vi "Periodic Tasks.vi"(8 "error in":errorcluster) -> ()   [LabVIEW 2013]
doc: "This VI runs in parallel to other tasks. It can contain as many user-defined periodic loops as you need. These can carry out PID or other sorts of timed response."
uses:
  GroundPassWrapperStates.ctl
  RefnameEnum.ctl
  CollectorWrapAction.ctl
  DoubleSolenoidAction.ctl
  <vilib>/Rock Robotics/WPI/Compressor/WPI_CompressorGetSetRefNum.vi
  Robot Global Data.vi
  <vilib>/Rock Robotics/SystemInterfaces/Utilities/FPGA_UtilitiesLED Source.ctl
  <vilib>/Rock Robotics/SystemInterfaces/Utilities/FPGA_UtilitiesLED State.ctl
  SingleSolenoidAction.ctl
  TankDriveAction.ctl
  ShooterWrapperAction.ctl
  SonarAction.ctl
  AutoAlignMode.ctl
  CatchAction.ctl
panel:
  out "GroundWrapperIterations":i32=2743
  out "GroundPassWrapper":u32=50
  in  "CollectorMotorSpeed":dbl=1.0
  out "AutoDistanceWrapperIterations":i32=6512
  out "AutoDistanceWrapperTimer":u32=20
  in  "Slowdown":dbl=12.0 format="%#_13g"
  in  "Brake":dbl=6.0 format="%#_13g"
  in  "DesiredDistance":dbl=144.0 format="%#_13g"
  out "CatcherWrapperIterations":i32=2744
  out "CatcherWrapperTimer":u32=50
  out "CollectorWrapperTimer":u32=50
  out "CollectorWrapperIterations":i32=2743
  out "ShooterWrapperIterations":i32=2667
  out "ShooterWrapperTimer":u32=50
  out "CollectorIterations":i32=2737
  out "ClapperIterations":i32=2743
  out "RollerPneumaticIterations":i32=2743
  out "RollerMotorIterations":i32=2742
  out "FiringCylinderIterations":i32=2745
  out "KickerIterations":i32=2744
  out "SonicShifterIterations":i32=2744
  out "TankDriveIterations":i32=6485
  out "Collector Timer":u32=50
  out "Clapper Timer":u32=50
  out "Roller Pneumatic Timer":u32=50
  out "Firing Cylinder Timer":u32=50
  out "Sonic Shifter Timer":u32=50
  out "Kicker Timer":u32=50
  out "Roller Motor Timer":u32=51
  out "Tank Drive Timer":u32=21
  # "CATCH"
  # "SHOOTER WRAP"
  # "SONIC SHIFTER"
  # "TANK DRIVE"
  # "COLLECTOR WRAP"
  # "KICKER"
  # "ROLLER MOTOR"
  # "COLLECTOR ARM"
  # "FIRING CYLINDERS"
  # "AUTODISTANCE"
  # "ROLLER PNEUMATIC"
  # "CLAPPER"
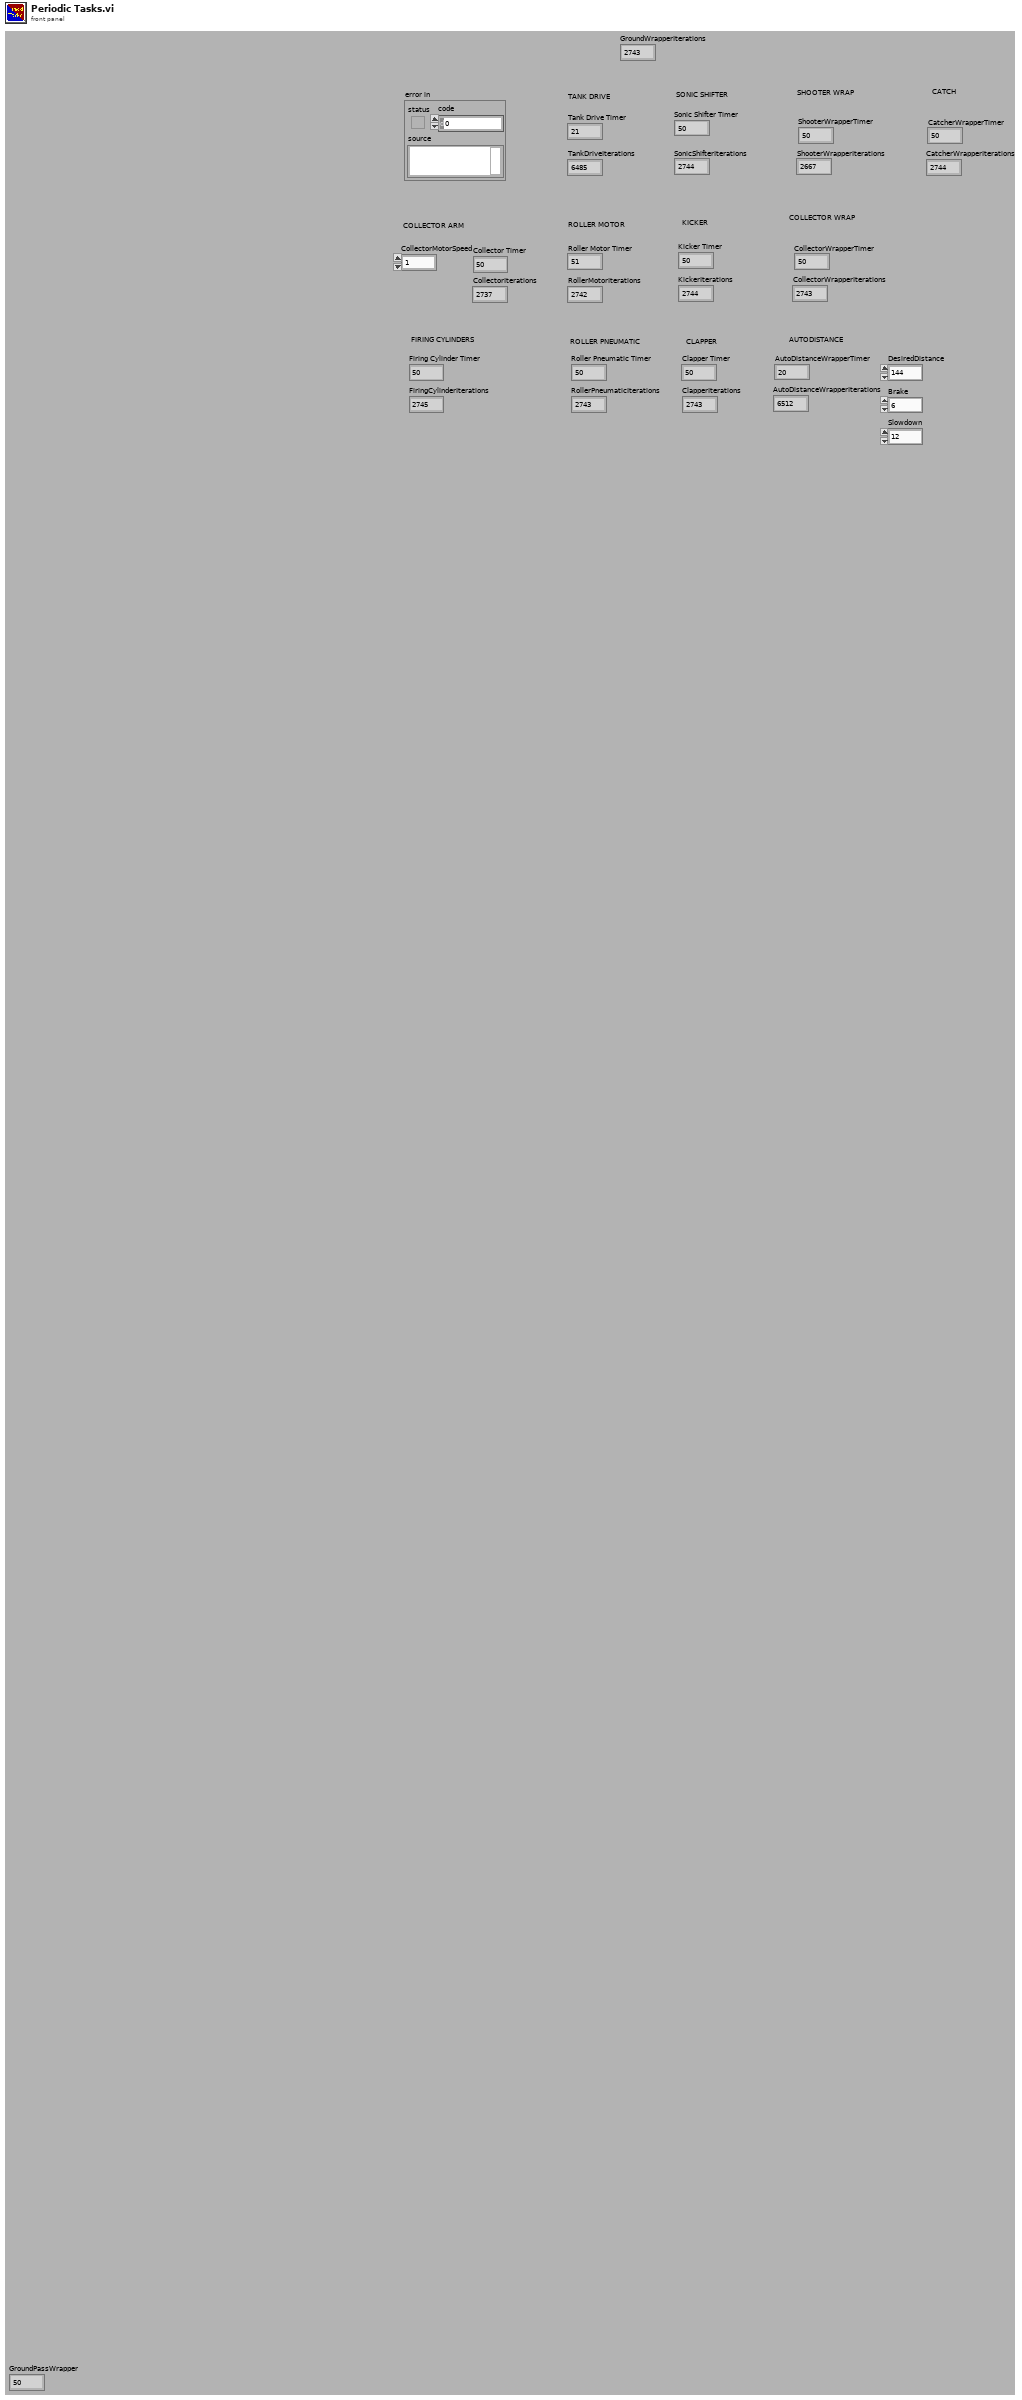
[diagram p1: front panel]
types:
  T1 = typedef "ShooterWrapperAction.ctl" = enum16{"Init", "CollectorDown", "CollectorUp"}
  T2 = typedef "CatchAction.ctl" = enum16{"PreCatch", "Catch", "Stop"}
  T3 = typedef "DoubleSolenoidAction.ctl" = enum16{"Init", "Middle", "In", "Out"}
  T4 = typedef "CollectorAction.ctl" = enum16{"Init", "Raise", "Lower", "Stop", "GetStatus"}
  T5 = typedef "CollectorWrapAction.ctl" = enum16{"PreCollect", "Collect", "Stop"}
  T6 = typedef "SingleSolenoidAction.ctl" = enum16{"Init", "SetState", "Disable"}
  T7 = typedef "TankDriveAction.ctl" = enum16{"Init", "LinearDrive", "SetValue", "Disable"}
  T8 = typedef "AutoAlignMode.ctl" = enum16{"Fullspeed", "Linear"}
  T9 = typedef "SonarAction.ctl" = enum16{"Init", "ReadValue", "Disable"}
  T10 = typedef "FPGA_UtilitiesLED State.ctl" = enum16{"Off", "On", "Toggle"}
  T11 = typedef "FPGA_UtilitiesLED Source.ctl" = enum16{"User LED", "FPGA LED"}
  T12 = typedef "RefnameEnum.ctl" = enum16{"TankDrive", "Controller1", "Controller2", "SonicShifter", "Compressor"}
  T13 = typedef "WPI_CompressorDevRef.ctl" = cluster{"DevStatus":errorcluster, "DigitalInputDevRef":T14, "RelayDevRef":T17}
  T14 = typedef "WPI_DigitalInputDevRef.ctl" = cluster{"DevStatus":errorcluster, "DIO Channel":T15, "Digital Module":T16}
  T15 = typedef "FPGA_DIOChannel.ctl" = enum8{"DIO 1", "DIO 2", "DIO 3", "DIO 4", "DIO 5", "DIO 6", "DIO 7", "DIO 8", "DIO 9", "DIO 10", "DIO 11", "DIO 12", "DIO 13", "DIO 14", "Invalid"}
  T16 = typedef "FPGA_TypedefDigitalModule.ctl" = enum16{"Digital Module 1", "Digital Module 2"}
  T17 = typedef "WPI_RelayDevRef.ctl" = cluster{"DevStatus":errorcluster, "Relay Channel":T18, "Digital Module":T16, "Relay Direction":T19}
  T18 = typedef "FPGA_DIORelayChannel.ctl" = enum8{"Relay 1", "Relay 2", "Relay 3", "Relay 4", "Relay 5", "Relay 6", "Relay 7", "Relay 8", "Invalid"}
  T19 = typedef "WPI_RelayDirection.ctl" = enum16{"Both directions", "Forward only", "Reverse only"}
  T20 = typedef "RollerAction.ctl" = enum16{"Init", "Off", "Forward", "Reverse"}
  T21 = typedef "GroundPassWrapperStates.ctl" = enum16{"Pass", "Stop"}
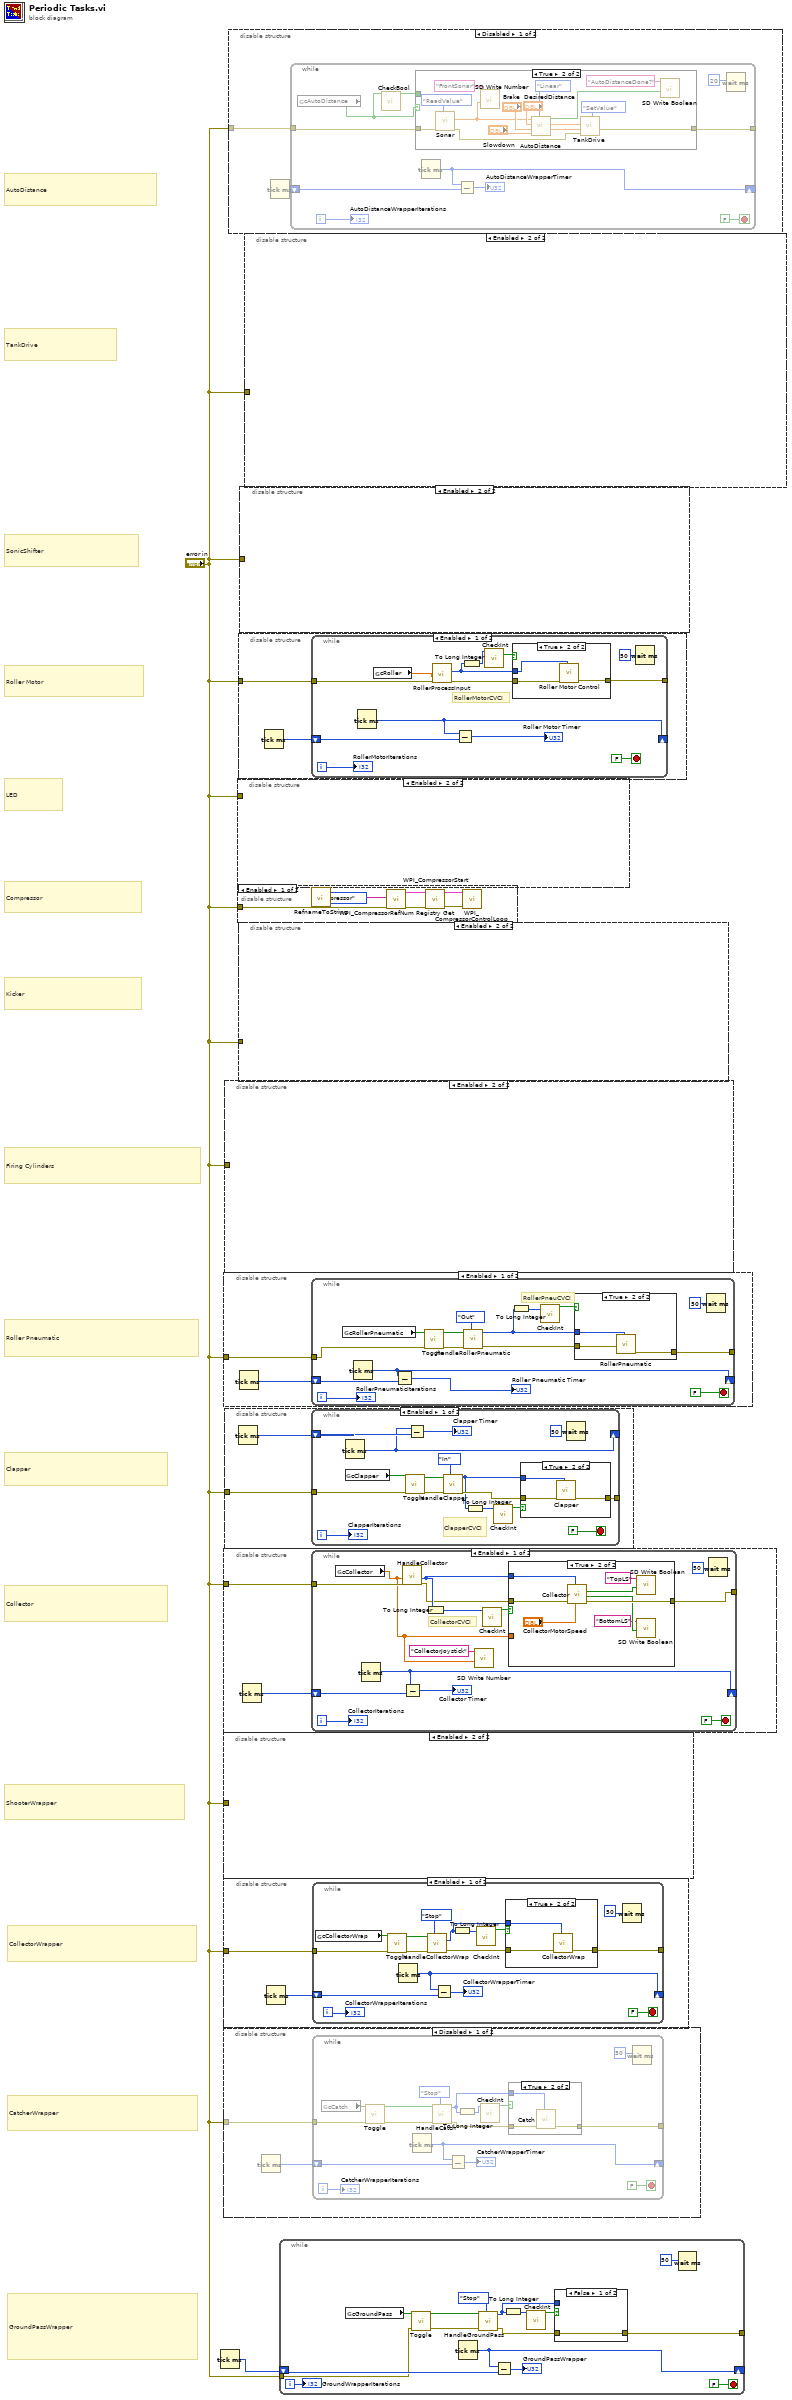
[diagram p0: block diagram]
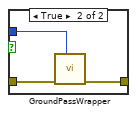
[diagram p2: hidden frame]
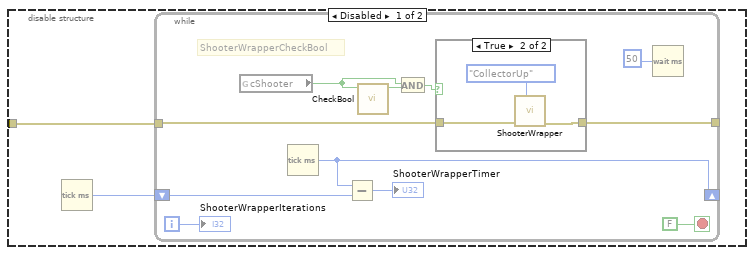
[diagram p7: hidden frame]
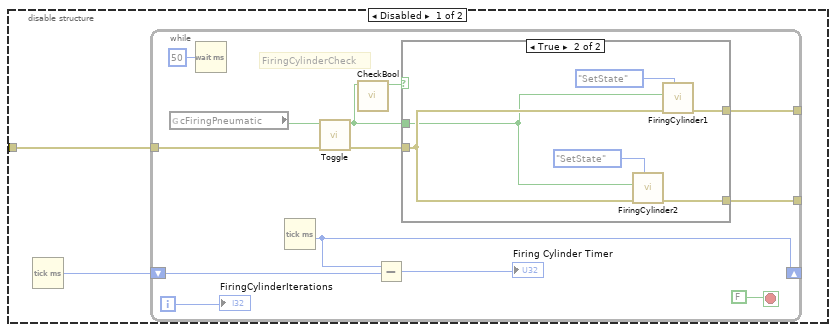
[diagram p15: hidden frame]
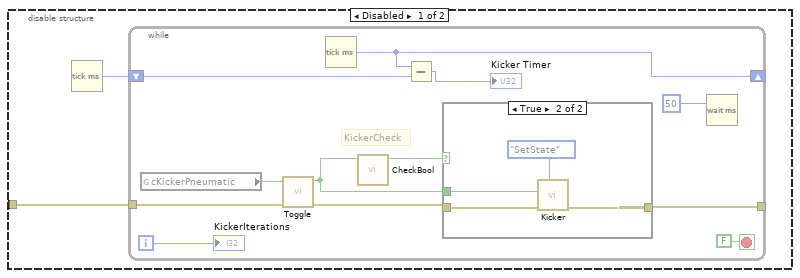
[diagram p17: hidden frame]
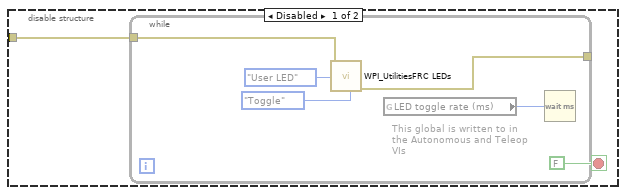
[diagram p20: hidden frame]
diagram:
  # "GroundPassWrapper"
  # "AutoDistance"
  # "CatcherWrapper"
  # "CollectorWrapper"
  # "ShooterWrapper"
  # "Collector"
  # "Clapper"
  # "Roller Pneumatic"
  # "Firing Cylinders"
  # "Kicker"
  # "Compressor"
  # "Roller Motor"
  # "SonicShifter"
  # "LED"
  # "TankDrive"
  n1 = Tick Count (ms)() -> (millisecond timer value=w1:u32)
  n2 = disable-structure shown="Enabled" {
    disable-tunnel: "error in" -> [w4 _]
    frame Disabled {
      n3 = Tick Count (ms)() -> (millisecond timer value=w3:u32)
      n4 = while {
        tunnel: w4 -> [w11]
        shift-right: [w12] -> _
        shift-left: w3 -> [w13]
        tunnel: [w10] -> _
        i -> [w8]
        stop <- FALSE stop-if-true
        # "ShooterWrapperCheckBool"
        n5 = global read "Robot Global Data.vi" "cShooter"() -> (w5:bool)
        n6 = Tick Count (ms)() -> (millisecond timer value=w12:u32)
        n7 = Subtract(x=w12, y=w13) -> (x-y=→"ShooterWrapperTimer":u32)
        n8 = call "CheckBool.vi"("Input Boolean"=w5) -> ("Boolean Changed?"=w7:bool)  [unwired: 10 in]
        n9 = And(x=w5, y=w7) -> (x .and. y?=w6:bool)
        n10 = case shown="True" w6 {
          tunnel: w11 -> [w16 w19]
          tunnel: [w16 w18] -> w10
          frame False {
          }
          frame True {
            n11 = call "ShooterWrapper.vi"("Action"=ShooterWrapperAction."CollectorUp", "error in"=w19) -> ("error out"=w18:errorcluster)  [unwired: 8 in]
          }
        }
        n12 = Wait (ms)(milliseconds to wait=u32 50) -> ()  [unwired: 1 out]
        "ShooterWrapperIterations" <- w8
      }
    }
    frame Enabled {
    }
  }
  n13 = disable-structure shown="Disabled" {
    disable-tunnel: "error in" -> [w21 _]
    frame Disabled {
      n14 = Tick Count (ms)() -> (millisecond timer value=w20:u32)
      n15 = while {
        tunnel: w21 -> [w37]
        tunnel: [w34] -> _
        shift-right: [w29] -> _
        shift-left: w20 -> [w30]
        i -> [w31]
        stop <- FALSE stop-if-true
        n16 = global read "Robot Global Data.vi" "cCatch"() -> (w36:bool)
        n17 = call "Toggle.vi"("error in"=w37, "RawInput"=w36) -> ("error out"=w27:errorcluster, "ToggleState"=w23:bool)  [unwired: 8 in]
        n18 = Tick Count (ms)() -> (millisecond timer value=w29:u32)
        n19 = call "HandleCatch.vi"("InitState"=CatchAction."Stop", "error in (no error)"=w27, "Toggle?"=w23) -> ("error out"=w26:errorcluster, "State"=w24:T2)  [unwired: 7 in]
        n20 = Subtract(x=w29, y=w30) -> (x-y=→"CatcherWrapperTimer":u32)
        n21 = To Long Integer(number=w24) -> (32bit integer=w25:i32)
        n22 = call "CheckInt.vi"("Integer"=w25) -> ("Changed?"=w35:bool)  [unwired: 10 in]
        n23 = case shown="True" w35 {
          tunnel: w26 -> [w38 w41]
          tunnel: [w38 w40] -> w34
          tunnel: w24 -> [_ w39]
          frame False {
          }
          frame True {
            n24 = call "Catch.vi"("Action"=w39, "error in (no error)"=w41) -> ("error out"=w40:errorcluster)  [unwired: 9 in]
          }
        }
        n25 = Wait (ms)(milliseconds to wait=u32 50) -> ()  [unwired: 1 out]
        "CatcherWrapperIterations" <- w31
      }
    }
    frame Enabled {
    }
  }
  n26 = disable-structure shown="Enabled" {
    disable-tunnel: "error in" -> [w43 _]
    frame Enabled {
      n27 = Tick Count (ms)() -> (millisecond timer value=w42:u32)
      n28 = while {
        tunnel: w43 -> [w47]
        shift-right: [w56] -> _
        shift-left: w42 -> [w55]
        tunnel: [w49] -> _
        i -> [w48]
        stop <- FALSE stop-if-true
        # "RollerPneuCVCI"
        n29 = global read "Robot Global Data.vi" "cRollerPneumatic"() -> (w45:bool)
        n30 = Tick Count (ms)() -> (millisecond timer value=w56:u32)
        n31 = Subtract(x=w56, y=w55) -> (x-y=→"Roller Pneumatic Timer":u32)
        n32 = call "Toggle.vi"("error in"=w47, "RawInput"=w45) -> ("error out"=w46:errorcluster, "ToggleState"=w44:bool)  [unwired: 8 in]
        n33 = call "HandleRollerPneumatic.vi"("InitState"=DoubleSolenoidAction."Out", "error in (no error)"=w46, "Toggle?"=w44) -> ("error out"=w50:errorcluster, "State"=w51:T3)  [unwired: 7 in]
        n34 = To Long Integer(number=w51) -> (32bit integer=w53:i32)
        n35 = call "CheckInt.vi"("Integer"=w53) -> ("Changed?"=w52:bool)  [unwired: 10 in]
        n36 = case shown="True" w52 {
          tunnel: w51 -> [_ w63]
          tunnel: w50 -> [w60 w62]
          tunnel: [w60 w61] -> w49
          frame False {
          }
          frame True {
            n37 = call "RollerPneumatic.vi"("State"=w63, "Error in"=w62) -> ("Error out"=w61:errorcluster)  [unwired: 9 in]
          }
        }
        n38 = Wait (ms)(milliseconds to wait=u32 50) -> ()  [unwired: 1 out]
        "RollerPneumaticIterations" <- w48
      }
    }
    frame Disabled {
    }
  }
  n39 = disable-structure shown="Enabled" {
    disable-tunnel: "error in" -> [w65 _]
    frame Enabled {
      n40 = Tick Count (ms)() -> (millisecond timer value=w64:u32)
      n41 = while {
        tunnel: w65 -> [w78]
        shift-right: [w75] -> _
        shift-left: w64 -> [w76]
        tunnel: [w69] -> _
        i -> [w68]
        stop <- FALSE stop-if-true
        # "CollectorCVCI"
        n42 = global read "Robot Global Data.vi" "cCollector"() -> (w66:dbl)
        n43 = Tick Count (ms)() -> (millisecond timer value=w75:u32)
        n44 = call "HandleCollector.vi"("error in"=w78, "JoystickValue"=w66) -> ("error out"=w70:errorcluster, "CollectorEnum Input"=w71:T4)  [unwired: 8 in]
        n45 = Subtract(x=w75, y=w76) -> (x-y=→"Collector Timer":u32)
        n46 = To Long Integer(number=w71) -> (32bit integer=w73:i32)
        n47 = call <vilib>:"SD Write Number.vi"("Numeric"=w66, "Name"="CollectorJoystick") -> ()  [unwired: 8 in, 2 out]
        n48 = call "CheckInt.vi"("Integer"=w73) -> ("Changed?"=w72:bool)  [unwired: 10 in]
        n49 = case shown="True" w72 {
          tunnel: w71 -> [_ w88]
          tunnel: w70 -> [w80 w87]
          tunnel: [w80 w86] -> w69
          tunnel: w66 -> [_ _]
          frame False {
          }
          frame True {
            n50 = call "Collector.vi"("MotorSpeed"="CollectorMotorSpeed", "Action"=w88, "Error in"=w87) -> ("Error out"=w86:errorcluster, "Lower Triggered?"=w84:bool, "Upper Triggered?"=w85:bool)  [unwired: 6 in]
            n51 = call <vilib>:"SD Write Boolean.vi"("Boolean"=w85, "Name"="TopLS") -> ()  [unwired: 8 in, 2 out]
            n52 = call <vilib>:"SD Write Boolean.vi"("Boolean"=w84, "Name"="BottomLS") -> ()  [unwired: 8 in, 2 out]
          }
        }
        n53 = Wait (ms)(milliseconds to wait=u32 50) -> ()  [unwired: 1 out]
        "CollectorIterations" <- w68
      }
    }
    frame Disabled {
    }
  }
  n54 = disable-structure shown="Enabled" {
    disable-tunnel: "error in" -> [w90 _]
    frame Enabled {
      n55 = Tick Count (ms)() -> (millisecond timer value=w89:u32)
      n56 = while {
        tunnel: w90 -> [w99]
        shift-right: [w103] -> _
        shift-left: w89 -> [w104]
        tunnel: [w102] -> _
        i -> [w100]
        stop <- FALSE stop-if-true
        n57 = global read "Robot Global Data.vi" "cCollectorWrap"() -> (w98:bool)
        n58 = call "Toggle.vi"("error in"=w99, "RawInput"=w98) -> ("error out"=w97:errorcluster, "ToggleState"=w95:bool)  [unwired: 8 in]
        n59 = Tick Count (ms)() -> (millisecond timer value=w103:u32)
        n60 = call "HandleCollectorWrap.vi"("InitState"=CollectorWrapAction."Stop", "error in (no error)"=w97, "Toggle?"=w95) -> ("error out"=w94:errorcluster, "State"=w91:T5)  [unwired: 7 in]
        n61 = Subtract(x=w103, y=w104) -> (x-y=→"CollectorWrapperTimer":u32)
        n62 = To Long Integer(number=w91) -> (32bit integer=w92:i32)
        n63 = call "CheckInt.vi"("Integer"=w92) -> ("Changed?"=w93:bool)  [unwired: 10 in]
        n64 = case shown="True" w93 {
          tunnel: [w107 w110] -> w102
          tunnel: w94 -> [w107 w109]
          tunnel: w91 -> [_ w108]
          frame False {
          }
          frame True {
            n65 = call "CollectorWrap.vi"("Action"=w108, "error in"=w109) -> ("error out"=w110:errorcluster)  [unwired: 9 in]
          }
        }
        n66 = Wait (ms)(milliseconds to wait=u32 50) -> ()  [unwired: 1 out]
        "CollectorWrapperIterations" <- w100
      }
    }
    frame Disabled {
    }
  }
  n67 = disable-structure shown="Enabled" {
    disable-tunnel: "error in" -> [w112 _]
    frame Disabled {
      n68 = Tick Count (ms)() -> (millisecond timer value=w111:u32)
      n69 = while {
        tunnel: w112 -> [w117]
        shift-right: [w123] -> _
        shift-left: w111 -> [w122]
        tunnel: [w120] -> _
        tunnel: [w119] -> _
        i -> [w113]
        stop <- FALSE stop-if-true
        # "FiringCylinderCheck"
        n70 = global read "Robot Global Data.vi" "cFiringPneumatic"() -> (w118:bool)
        n71 = Wait (ms)(milliseconds to wait=u32 50) -> ()  [unwired: 1 out]
        n72 = Tick Count (ms)() -> (millisecond timer value=w123:u32)
        n73 = call "Toggle.vi"("error in"=w117, "RawInput"=w118) -> ("error out"=w116:errorcluster, "ToggleState"=w114:bool)  [unwired: 8 in]
        n74 = call "CheckBool.vi"("Input Boolean"=w114) -> ("Boolean Changed?"=w115:bool)  [unwired: 10 in]
        n75 = Subtract(x=w123, y=w122) -> (x-y=→"Firing Cylinder Timer":u32)
        n76 = case shown="True" w115 {
          tunnel: w116 -> [w126 w128]
          tunnel: [w126 w130] -> w120
          tunnel: [w126 w129] -> w119
          tunnel: w114 -> [_ w127]
          frame False {
          }
          frame True {
            n77 = call "FiringCylinder2.vi"("Action"=SingleSolenoidAction."SetState", "error in (no error)"=w128, "Actuate?"=w127) -> ("error out"=w129:errorcluster)  [unwired: 8 in]
            n78 = call "FiringCylinder1.vi"("Action"=SingleSolenoidAction."SetState", "error in (no error)"=w128, "Actuate?"=w127) -> ("error out"=w130:errorcluster)  [unwired: 8 in]
          }
        }
        "FiringCylinderIterations" <- w113
      }
    }
    frame Enabled {
    }
  }
  n79 = disable-structure shown="Enabled" {
    disable-tunnel: "error in" -> [w134 _]
    frame Enabled {
      n80 = Tick Count (ms)() -> (millisecond timer value=w133:u32)
      n81 = while {
        tunnel: w134 -> [w139]
        shift-right: [w135] -> _
        shift-left: w133 -> [w136]
        tunnel: [w145] -> _
        i -> [w141]
        stop <- FALSE stop-if-true
        # "ClapperCVCI"
        n82 = Tick Count (ms)() -> (millisecond timer value=w135:u32)
        n83 = global read "Robot Global Data.vi" "cClapper"() -> (w140:bool)
        n84 = call "Toggle.vi"("error in"=w139, "RawInput"=w140) -> ("error out"=w138:errorcluster, "ToggleState"=w137:bool)  [unwired: 8 in]
        n85 = Subtract(x=w135, y=w136) -> (x-y=→"Clapper Timer":u32)
        n86 = call "HandleClapper.vi"("InitState"=DoubleSolenoidAction."In", "error in (no error)"=w138, "Toggle?"=w137) -> ("error out"=w146:errorcluster, "State"=w143:T3)  [unwired: 7 in]
        n87 = To Long Integer(number=w143) -> (32bit integer=w144:i32)
        n88 = call "CheckInt.vi"("Integer"=w144) -> ("Changed?"=w142:bool)  [unwired: 10 in]
        n89 = case shown="True" w142 {
          tunnel: w143 -> [_ w154]
          tunnel: w146 -> [w151 w153]
          tunnel: [w151 w152] -> w145
          frame False {
          }
          frame True {
            n90 = call "Clapper.vi"("State"=w154, "Error in"=w153) -> ("Error out"=w152:errorcluster)  [unwired: 9 in]
          }
        }
        n91 = Wait (ms)(milliseconds to wait=u32 50) -> ()  [unwired: 1 out]
        "ClapperIterations" <- w141
      }
    }
    frame Disabled {
    }
  }
  n92 = disable-structure shown="Disabled" {
    disable-tunnel: "error in" -> [w156 _]
    frame Disabled {
      n93 = Tick Count (ms)() -> (millisecond timer value=w155:u32)
      n94 = while {
        tunnel: w156 -> [w166]
        tunnel: [w165] -> _
        shift-right: [w160] -> _
        shift-left: w155 -> [w161]
        i -> [w162]
        stop <- FALSE stop-if-true
        n95 = global read "Robot Global Data.vi" "cAutoDistance"() -> (w158:bool)
        n96 = call "CheckBool.vi"("Input Boolean"=w158) -> ("Boolean Changed?"=w157:bool)  [unwired: 10 in]
        n97 = case shown="True" w158 {
          tunnel: w166 -> [w169 w185]
          tunnel: [w168 w182] -> w165
          tunnel: w157 -> [w167 _]
          frame False {
            n98 = case shown="True" w167 {
              tunnel: w169 -> [w170 w174]
              tunnel: [w170 w173] -> w168
              frame False {
              }
              frame True {
                w172 = 0.0 ("LeftDesired")
                n99 = call "TankDrive.vi"("DriveAction"=TankDriveAction."SetValue", "error in (no error)"=w174, "RightDesired"=w172, "LeftDesired"=w172) -> ("error out"=w173:errorcluster)  [unwired: 6 in, 1 out]
              }
            }
          }
          frame True {
            n100 = call "Sonar.vi"("Action"=SonarAction."ReadValue", "error in (no error)"=w185) -> ("error out"=w179:errorcluster, "distance"=w181:dbl)  [unwired: 8 in]
            n101 = call <vilib>:"SD Write Number.vi"("Numeric"=w181, "Name"="FrontSonar") -> ()  [unwired: 8 in, 2 out]
            n102 = call "AutoDistance.vi"("Mode"=AutoAlignMode."Linear", "Slowdown"="Slowdown", "Brake"="Brake", "DesiredDistance"="DesiredDistance", "CurrentDistance"=w181) -> ("TankDriveRight"=w175:dbl, "TankDriveLeft"=w176:dbl, "Finished"=w178:bool)  [unwired: 4 in]
            n103 = call "TankDrive.vi"("DriveAction"=TankDriveAction."SetValue", "error in (no error)"=w179, "RightDesired"=w175, "LeftDesired"=w176) -> ("error out"=w182:errorcluster)  [unwired: 6 in, 1 out]
            n104 = call <vilib>:"SD Write Boolean.vi"("Boolean"=w178, "Name"="AutoDistanceDone?") -> ()  [unwired: 8 in, 2 out]
          }
        }
        n105 = Tick Count (ms)() -> (millisecond timer value=w160:u32)
        n106 = Subtract(x=w160, y=w161) -> (x-y=→"AutoDistanceWrapperTimer":u32)
        n107 = Wait (ms)(milliseconds to wait=u32 20) -> ()  [unwired: 1 out]
        "AutoDistanceWrapperIterations" <- w162
      }
    }
    frame Enabled {
    }
  }
  n108 = disable-structure shown="Enabled" {
    disable-tunnel: "error in" -> [w190 _]
    frame Disabled {
      n109 = while {
        tunnel: w190 -> [w192]
        tunnel: [w191] -> _
        stop <- FALSE stop-if-true
        # "This global is written to in the Autonomous and Teleop VIs"
        n110 = call <vilib>:"WPI_UtilitiesFRC LEDs.vi"("error in (no error)"=w192, "State"=FPGA_UtilitiesLED_State."Toggle", "LED Type"=FPGA_UtilitiesLED_Source."User LED") -> ("error out"=w191:errorcluster)  [unwired: 8 out]
        n111 = global read "Robot Global Data.vi" "LED toggle rate (ms)"() -> (w193:u32)
        n112 = Wait (ms)(milliseconds to wait=w193) -> ()  [unwired: 1 out]
      }
    }
    frame Enabled {
    }
  }
  n113 = disable-structure shown="Enabled" {
    disable-tunnel: "error in" -> [w203 _]
    frame Enabled {
      n114 = call "RefnameToString.vi"("Enum"=RefnameEnum."Compressor") -> ("Refname"=w200:string)
      n115 = call <vilib>:"WPI_CompressorRefNum Registry Get.vi"("error in (no error)"=w203, "refnum name"=w200) -> ("error out"=w202:errorcluster, "CompressorDevRef"=w198:T13)  [unwired: 8 in]
      n116 = call <vilib>:"WPI_CompressorStart.vi"("error in (no error)"=w202, "CompressorDevRef"=w198) -> ("error out"=w201:errorcluster, "CompressorDevRef"=w197:T13)  [unwired: 8 in]
      n117 = call <vilib>:"WPI_CompressorControlLoop.vi"("error in (no error)"=w201, "CompressorDevRef"=w197) -> ()  [unwired: 10 in]
    }
    frame Disabled {
    }
  }
  n118 = disable-structure shown="Enabled" {
    disable-tunnel: "error in" -> [w205 _]
    frame Enabled {
      n119 = Tick Count (ms)() -> (millisecond timer value=w204:u32)
      n120 = while {
        tunnel: w205 -> [w216]
        shift-right: [w214] -> _
        shift-left: w204 -> [w212]
        tunnel: [w208] -> _
        i -> [w206]
        stop <- FALSE stop-if-true
        # "RollerMotorCVCI"
        n121 = Tick Count (ms)() -> (millisecond timer value=w214:u32)
        n122 = global read "Robot Global Data.vi" "cRoller"() -> (w215:dbl)
        n123 = call "RollerProcessInput.vi"("error in"=w216, "JoystickValue"=w215) -> ("error out"=w209:errorcluster, "StateOut"=w207:T20)  [unwired: 8 in]
        n124 = Subtract(x=w214, y=w212) -> (x-y=→"Roller Motor Timer":u32)
        n125 = To Long Integer(number=w207) -> (32bit integer=w211:i32)
        n126 = call "CheckInt.vi"("Integer"=w211) -> ("Changed?"=w210:bool)  [unwired: 10 in]
        n127 = case shown="True" w210 {
          tunnel: w207 -> [_ w222]
          tunnel: w209 -> [w219 w221]
          tunnel: [w219 w220] -> w208
          frame False {
          }
          frame True {
            n128 = call "Roller Motor Control.vi"("Action"=w222, "Error in"=w221) -> ("Error out"=w220:errorcluster)  [unwired: 9 in]
          }
        }
        n129 = Wait (ms)(milliseconds to wait=u32 50) -> ()  [unwired: 1 out]
        "RollerMotorIterations" <- w206
      }
    }
    frame Disabled {
    }
  }
  n130 = disable-structure shown="Enabled" {
    disable-tunnel: "error in" -> [w224 _]
    frame Disabled {
      n131 = Tick Count (ms)() -> (millisecond timer value=w223:u32)
      n132 = while {
        tunnel: w224 -> [w230]
        shift-right: [w232] -> _
        shift-left: w223 -> [w234]
        tunnel: [w231] -> _
        i -> [w225]
        stop <- FALSE stop-if-true
        # "KickerCheck"
        n133 = global read "Robot Global Data.vi" "cKickerPneumatic"() -> (w228:bool)
        n134 = call "Toggle.vi"("error in"=w230, "RawInput"=w228) -> ("error out"=w229:errorcluster, "ToggleState"=w226:bool)  [unwired: 8 in]
        n135 = Tick Count (ms)() -> (millisecond timer value=w232:u32)
        n136 = call "CheckBool.vi"("Input Boolean"=w226) -> ("Boolean Changed?"=w227:bool)  [unwired: 10 in]
        n137 = Subtract(x=w232, y=w234) -> (x-y=→"Kicker Timer":u32)
        n138 = case shown="True" w227 {
          tunnel: w229 -> [w237 w239]
          tunnel: [w237 w240] -> w231
          tunnel: w226 -> [_ w238]
          frame False {
          }
          frame True {
            n139 = call "Kicker.vi"("Action"=SingleSolenoidAction."SetState", "error in (no error)"=w239, "Actuate?"=w238) -> ("error out"=w240:errorcluster)  [unwired: 8 in]
          }
        }
        n140 = Wait (ms)(milliseconds to wait=u32 50) -> ()  [unwired: 1 out]
        "KickerIterations" <- w225
      }
    }
    frame Enabled {
    }
  }
  n141 = disable-structure shown="Enabled" {
    disable-tunnel: "error in" -> [w243 _]
    frame Disabled {
      n142 = Tick Count (ms)() -> (millisecond timer value=w242:u32)
      n143 = while {
        tunnel: w243 -> [w248]
        shift-right: [w252] -> _
        shift-left: w242 -> [w253]
        tunnel: [w250] -> _
        i -> [w245]
        stop <- FALSE stop-if-true
        n144 = global read "Robot Global Data.vi" "cSonicShifter"() -> (w249:bool)
        n145 = call "Toggle.vi"("error in"=w248, "RawInput"=w249) -> ("error out"=w247:errorcluster, "ToggleState"=w244:bool)  [unwired: 8 in]
        n146 = Tick Count (ms)() -> (millisecond timer value=w252:u32)
        n147 = Subtract(x=w252, y=w253) -> (x-y=→"Sonic Shifter Timer":u32)
        n148 = call "CheckBool.vi"("Input Boolean"=w244) -> ("Boolean Changed?"=w246:bool)  [unwired: 10 in]
        n149 = case shown="True" w246 {
          tunnel: [w256 w259] -> w250
          tunnel: w247 -> [w256 w258]
          tunnel: w244 -> [_ w257]
          frame False {
          }
          frame True {
            n150 = call "SonicShifter.vi"("Action"=SingleSolenoidAction."SetState" ("Mode"), "error in (no error)"=w258, "Actuate?"=w257) -> ("error out"=w259:errorcluster)  [unwired: 8 in]
          }
        }
        n151 = Wait (ms)(milliseconds to wait=u32 50) -> ()  [unwired: 1 out]
        "SonicShifterIterations" <- w245
      }
    }
    frame Enabled {
    }
  }
  n152 = disable-structure shown="Enabled" {
    disable-tunnel: "error in" -> [w262 _]
    frame Disabled {
      n153 = Tick Count (ms)() -> (millisecond timer value=w261:u32)
      n154 = while {
        tunnel: w262 -> [w267]
        shift-right: [w286] -> _
        shift-left: w261 -> [w285]
        tunnel: [w278] -> _
        i -> [w275]
        stop <- FALSE stop-if-true
        n155 = global read "Robot Global Data.vi" "cReverseDrive"() -> (w274:bool)
        n156 = global read "Robot Global Data.vi" "cStraightDrive"() -> (w271:bool)
        n157 = global read "Robot Global Data.vi" "cTankDriveRight"() -> (w283:dbl)
        n158 = global read "Robot Global Data.vi" "cTankDriveLeft"() -> (w282:dbl)
        n159 = global read "Robot Global Data.vi" "cHalfDrive"() -> (w270:bool)
        n160 = Tick Count (ms)() -> (millisecond timer value=w286:u32)
        n161 = Wait (ms)(milliseconds to wait=u32 20) -> ()  [unwired: 1 out]
        n162 = call "Toggle.vi"("RawInput"=w274) -> ("ToggleState"=w268:bool)  [unwired: 9 in, 1 out]
        n163 = Subtract(x=w286, y=w285) -> (x-y=→"Tank Drive Timer":u32)
        n164 = call "Sonar.vi"("Action"=SonarAction."ReadValue", "error in (no error)"=w267) -> ("error out"=w265:errorcluster, "distance"=w263:dbl)  [unwired: 8 in]
        n165 = call "HandleDrive.vi"("Deadzone"=0.15, "RightMotor"=w283, "LeftMotor"=w282) -> ("Enqueue?"=w281:bool, "RightMotor"=w279:dbl, "LeftMotor"=w280:dbl)  [unwired: 6 in]
        n166 = call <vilib>:"SD Write Boolean.vi"("Boolean"=w268, "Name"="ReverseDrive") -> ()  [unwired: 8 in, 2 out]
        n167 = call <vilib>:"SD Write Number.vi"("error in"=w265, "Numeric"=w263, "Name"="FrontSonar") -> ()  [unwired: 7 in, 2 out]
        n168 = call <vilib>:"SD Write Boolean.vi"("Boolean"=w271, "Name"="StraightDrive") -> ()  [unwired: 8 in, 2 out]
        n169 = call <vilib>:"SD Write Boolean.vi"("Boolean"=w270, "Name"="HalfDrive") -> ()  [unwired: 8 in, 2 out]
        n170 = case shown="True" w281 {
          tunnel: w280 -> [_ w297]
          tunnel: w279 -> [_ w296]
          tunnel: [w288 w295] -> w278
          tunnel: w267 -> [w288 w294]
          tunnel: w268 -> [_ w291]
          tunnel: w270 -> [_ w290]
          tunnel: w271 -> [_ w289]
          frame False {
          }
          frame True {
            w304 = 0.0  # Cutoff
            n171 = call "HalfDrive.vi"("RightDrive in"=w296, "LeftDrive in"=w297, "HalfDrive"=w290) -> ("RightDrive out"=w303:dbl, "LeftDrive out"=w302:dbl)  [unwired: 7 in]
            n172 = call "StraightDrive.vi"("RightDrive in"=w303, "LeftDrive in"=w302, "StraightDrive"=w289) -> ("RightDrive out"=w300:dbl, "LeftDrive out"=w301:dbl)  [unwired: 7 in]
            n173 = call "ReverseDrive.vi"("cReverseDrive"=w291, "Right"=w300, "Left"=w301) -> ("Right"=w298:dbl, "Left"=w299:dbl)  [unwired: 7 in]
            n174 = call <vilib>:"SD Read Number.vi"("Name"="MaxMotorChange") -> ("Numeric"=w292:dbl)  [unwired: 8 in, 2 out]
            n175 = call "TankDrive.vi"("MaxMotorChangeForward"=w292, "Cutoff"=w304, "DriveAction"=TankDriveAction."SetValue", "error in (no error)"=w294, "RightDesired"=w298, "LeftDesired"=w299) -> ("error out"=w295:errorcluster)  [unwired: 4 in, 1 out]
          }
        }
        "TankDriveIterations" <- w275
      }
    }
    frame Enabled {
    }
  }
  n176 = while {
    tunnel: "error in" -> [w310]
    shift-right: [w311] -> _
    shift-left: w1 -> [w312]
    tunnel: [w309] -> _
    i -> [w308]
    stop <- FALSE stop-if-true
    n177 = global read "Robot Global Data.vi" "cGroundPass"() -> (w320:bool)
    n178 = call "Toggle.vi"("error in"=w310, "RawInput"=w320) -> ("error out"=w316:errorcluster, "ToggleState"=w313:bool)  [unwired: 8 in]
    n179 = Tick Count (ms)() -> (millisecond timer value=w311:u32)
    n180 = call "HandleGroundPass.vi"("InitState"=GroundPassWrapperStates."Stop", "error in"=w316, "Toggle?"=w313) -> ("error out"=w315:errorcluster, "State"=w306:T21)  [unwired: 7 in]
    n181 = Subtract(x=w311, y=w312) -> (x-y=→"GroundPassWrapper":u32)
    n182 = To Long Integer(number=w306) -> (32bit integer=w314:i32)
    n183 = call "CheckInt.vi"("Integer"=w314) -> ("Changed?"=w319:bool)  [unwired: 10 in]
    n184 = case shown="False" w319 {
      tunnel: w315 -> [w322 w325]
      tunnel: [w322 w324] -> w309
      tunnel: w306 -> [_ w323]
      frame False {
      }
      frame True {
        n185 = call "GroundPassWrapper.vi"("State"=w323, "error in"=w325) -> ("error out"=w324:errorcluster)  [unwired: 9 in]
      }
    }
    n186 = Wait (ms)(milliseconds to wait=u32 50) -> ()  [unwired: 1 out]
    "GroundWrapperIterations" <- w308
  }
